vi "GRPCServerExample.vi"() -> ()   [LabVIEW 2019, in "MicronGRPCServer.lvlib"]
uses:
  Service/MicronGRPCServer.lvlib
  Base/Server/Service/ServiceBase.lvclass
  Base/Server/Message/MessageBase.lvclass
  <vilib>/SLL Toolkit/SLL String/SLL String.lvlib
  Service/GRPCService.lvclass
panel:
  in  "Stop":bool
  in  "Connection String":string="localhost:50051"
  out "Last Message Timestamp":string
  out "Payload":string
  out "Command":string
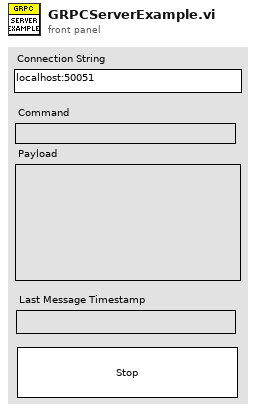
[diagram p1: front panel]
types:
  T1 = typedef "MicronServer.lvlib/ServiceBase.lvclass/Micron Args.ctl" = cluster{"Network":string, "Name":string, "Port":i32, "Connection":string, "Args":string[], "Alias":string}
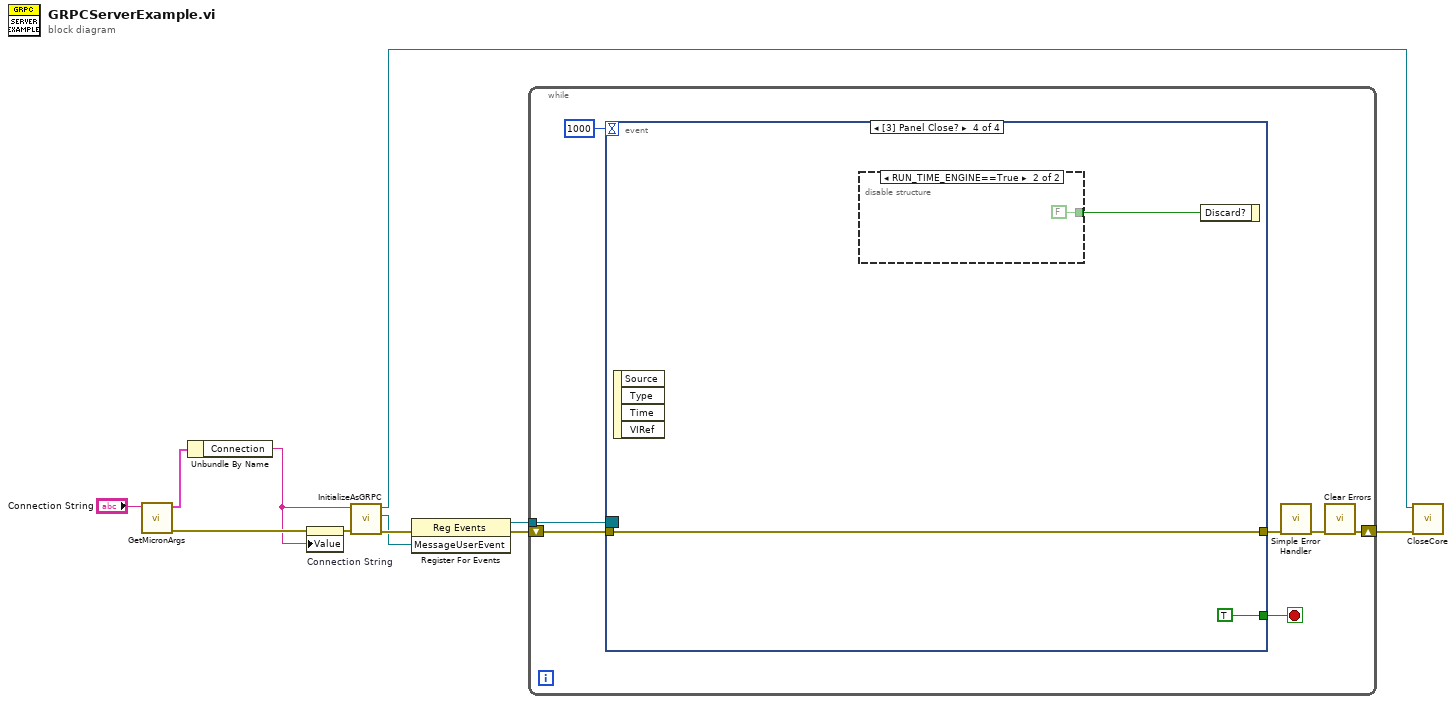
[diagram p0: block diagram]
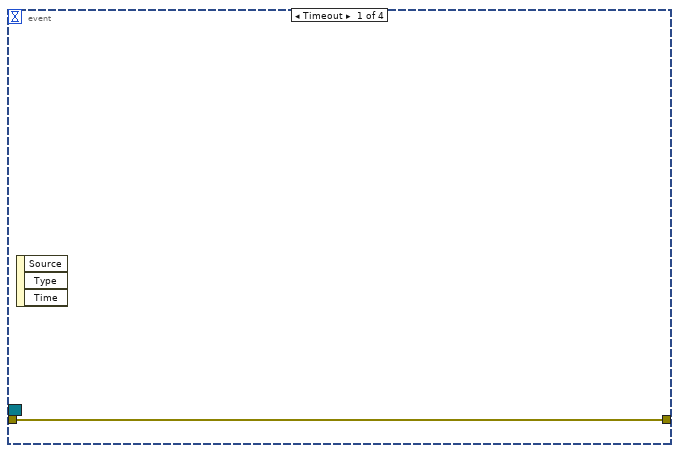
[diagram p2: hidden frame]
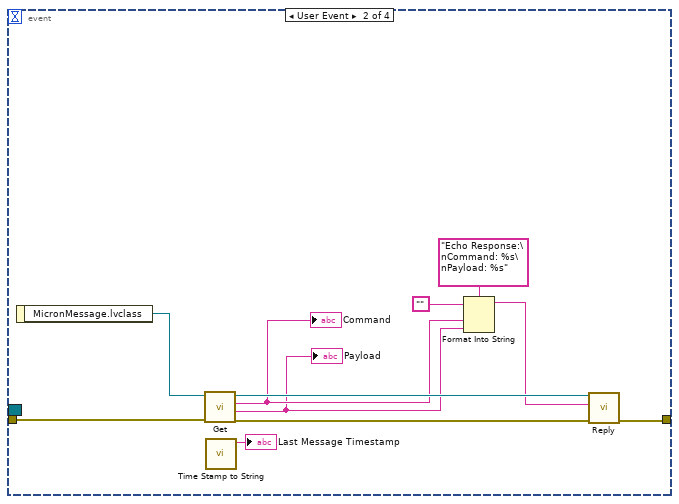
[diagram p3: hidden frame]
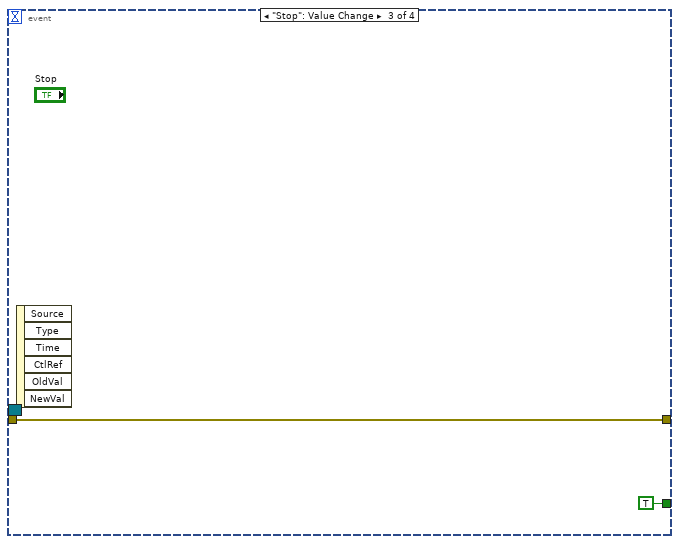
[diagram p4: hidden frame]
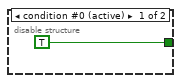
[diagram p5: hidden frame]
diagram:
  n1 = call "GetMicronArgs.vi"("Default Connection String"="Connection String") -> ("error out"=w4:errorcluster, "Micron Args"=w3:T1)  [unwired: 9 in]
  n2 = Unbundle By Name(w3) -> ("Connection"=w1:string)
  n3 = property on="Connection String" class="Str"(error in=w4, "Value"=w1) -> (error out=w5:errorcluster)  [unwired: 1 in, 1 out]
  n4 = call "InitializeAsGRPC.vi"("error in (no error)"=w5, "Connection String"=w1) -> ("error out"=w11:errorcluster, "MessageUserEvent"=w7:refnum<user-event>, "MicronServer"=w6:refnum<class "ServiceBase.lvclass">)  [unwired: 7 in]
  n5 = register-events(error in=w11, w7) -> (reference out=w10:refnum<event-registration>, error out=w9:errorcluster)  [unwired: 1 in]
  n6 = while {
    tunnel: w10 -> [w16]
    shift-right: [w12] -> w8
    shift-left: w9 -> [w15]
    stop <- w17 stop-if-true
    n7 = event shown="[3] Panel Close?" {
      selector: w16 -> [_ _ _ _]
      dyn-events: _ -> [_ _ _ _]
      timeout: 1000 -> [_ _ _ _]
      tunnel: [w19 w27 w32 w33] -> w14
      tunnel: [_ _ TRUE TRUE] -> w17
      tunnel: w15 -> [w19 w20 w32 w33]
      event Timeout {
        n8 = event-data() -> ()  [unwired: 1 in, 3 out]
      }
      event User Event {
        n9 = event-data() -> ("MicronMessage.lvclass"=w30:refnum<class "MessageBase.lvclass">)  [unwired: 1 in]
        n10 = call-dynamic "Get.vi"("error in (no error)"=w20, "MicronMessage in"=w30) -> ("error out"=w29:errorcluster, "Payload"=w24:string, "Command"=w25:string, "MicronMessage out"=w28:refnum<class "MessageBase.lvclass">)  [unwired: 6 in]
        "Command" <- w25
        "Payload" <- w24
        n11 = call <vilib>:"Time Stamp to String.vi"() -> ("Output String"=→"Last Message Timestamp":string)  [unwired: 11 in]
        n12 = Format Into String(format string="Echo Response:\nCommand: %s\nPayload: %s", initial string="", w25, w24) -> (resulting string=w22:string)  [unwired: 1 in, 1 out]
        n13 = call-dynamic "Reply.vi"("error in (no error)"=w29, "Response"=w22, "MicronMessage in"=w28) -> ("error out"=w27:errorcluster)  [unwired: 7 in, 1 out]
      }
      event "Stop": Value Change {
        n14 = event-data() -> ()  [unwired: 1 in, 6 out]
      }
      event Panel Close? {
        n15 = event-data() -> ()  [unwired: 1 in, 4 out]
        n16 = disable-structure shown="RUN_TIME_ENGINE==True" {
          disable-tunnel: [TRUE ("Discard?") FALSE ("Discard?")] -> w35
          frame condition #0 (active) {
          }
          frame condition #1 {
          }
        }
        n17 = event-data("Discard?"=w35) -> ()  [unwired: 1 in, 1 out]
      }
    }
    n18 = call <vilib>:"Simple Error Handler.vi"("error in (no error)"=w14) -> ("error out"=w13:errorcluster)  [unwired: 4 in, 4 out]
    n19 = call <vilib>:"Clear Errors.vi"("error in (no error)"=w13) -> ("error out"=w12:errorcluster)  [unwired: 5 in, 1 out]
  }
  n20 = call-dynamic "CloseCore.vi"("error in (no error)"=w8, "MicronServer in"=w6) -> ()  [unwired: 8 in, 2 out]
